vi "Facade - impuls graph.vi"(0 "Data In":T4, 2 "Display State In":T2, 3 "Container State":T3) -> (6 "Data Out":T4, 7 "Display State Out":T2, 8 "Action":T1)   [LabVIEW 2016, in "impuls graph.xctl"]
uses:
  impuls graph.xctl
  Data - impuls graph.ctl
  <vilib>/_xctls/Container State.ctl
  State - impuls graph.ctl
  <vilib>/_xctls/Action.ctl
  <vilib>/_xctls/XControlSupport.lvlib
panel:
  out "Waveform Graph":dbl[][](graph)
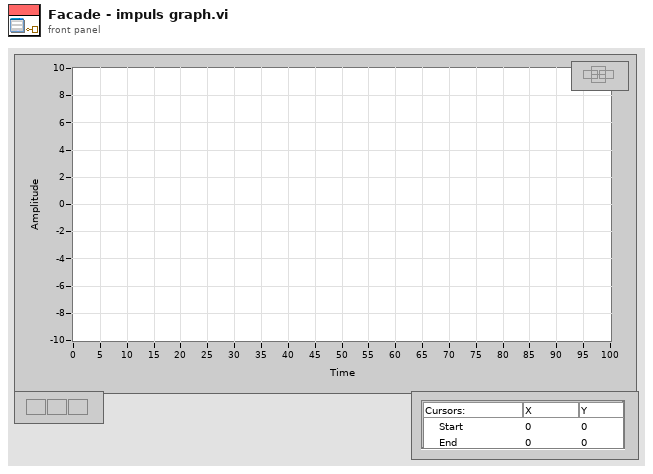
[diagram p1: front panel]
types:
  T1 = typedef "XControlSupport.lvlib/Action.ctl" = cluster{"Data Changed?":bool, "State Changed?":bool, "Action Name":string}
  T2 = typedef "impuls graph.xctl/State - impuls graph.ctl" = cluster{"Waveform Graph":refnum<vi>}
  T3 = typedef "XControlSupport.lvlib/Container State.ctl" = cluster{"Indicator?":bool, "Run Mode?":bool, " Refnum":refnum<vi>}
  T4 = typedef "impuls graph.xctl/Data - impuls graph.ctl" = cluster{"Data":dbl[][], "Colour":u32, "Channel Name":string, "Sample Rate":dbl, "Visible":bool}[]
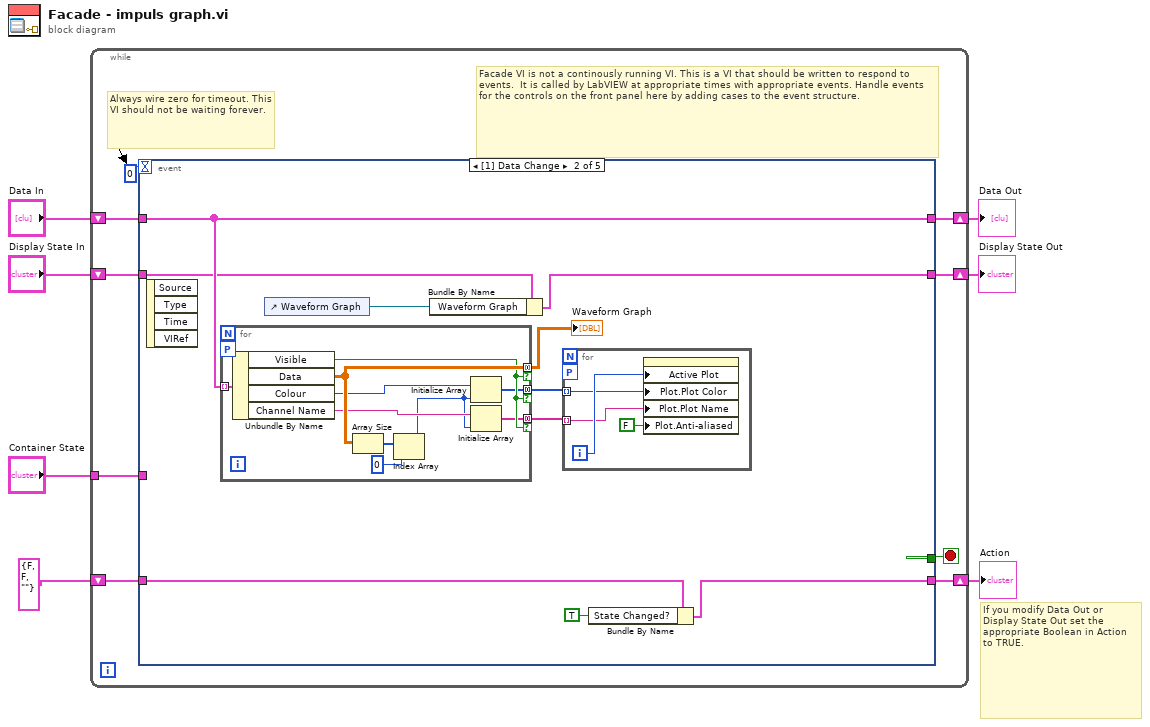
[diagram p0: block diagram]
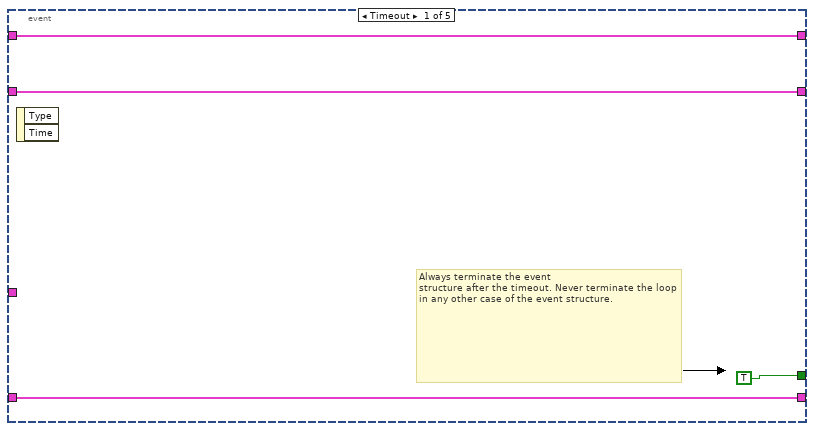
[diagram p2: hidden frame]
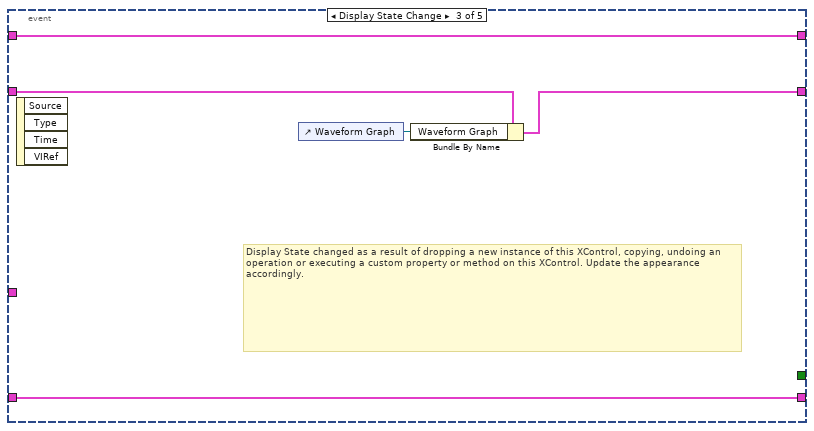
[diagram p3: hidden frame]
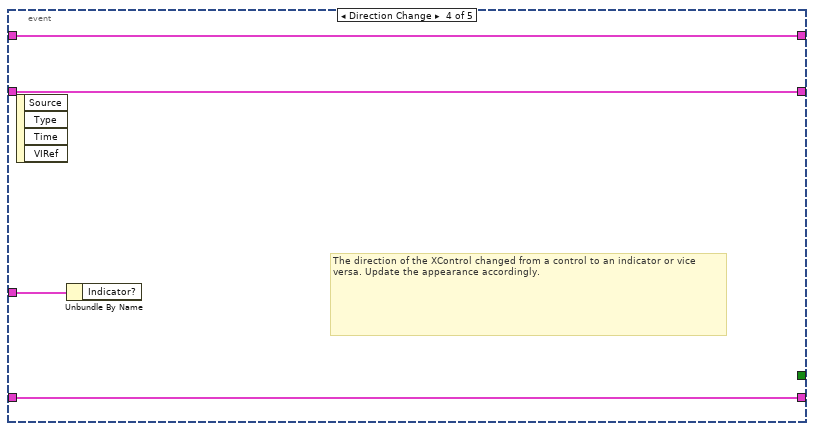
[diagram p4: hidden frame]
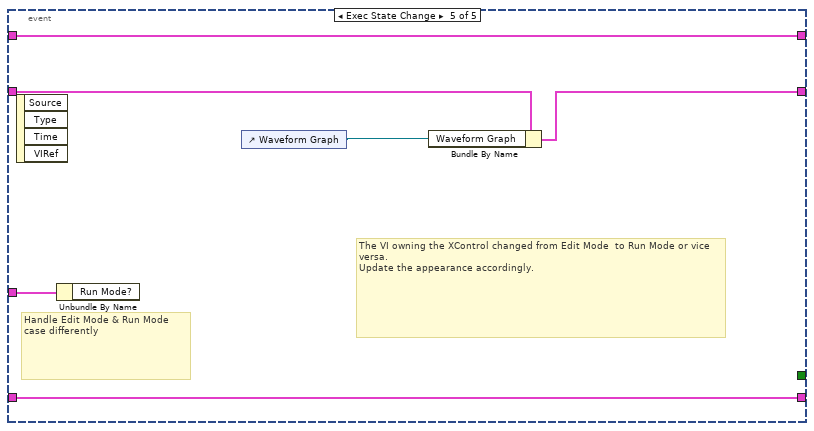
[diagram p5: hidden frame]
diagram:
  # "If you modify Data Out or\nDisplay State Out set the\nappropriate Boolean in Action\nto TRUE."
  n1 = while {
    shift-right: [w15] -> w4
    shift-left: "Display State In" -> [w16]
    tunnel: "Container State" -> [w12]
    shift-right: [w10] -> w7
    shift-left: "Data In" -> [w11]
    shift-right: [w8] -> w2
    shift-left: T1 {"Data Changed?"=FALSE, "State Changed?"=FALSE, "Action Name"=""} ("Action") -> [w9]
    stop <- w14 stop-if-true
    # "Facade VI is not a continously running VI. This is a VI that should be written to respond to events.  It is called by LabVIEW at appropriate times with appropriate events. Handle events for the controls on the front panel here by adding cases to the event structure."
    # "Always wire zero for timeout. This\nVI should not be waiting forever."
    n2 = event shown="[1] Data Change" {
      selector: _ -> [_ _ _ _ _]
      dyn-events: _ -> [_ _ _ _ _]
      timeout: 0 -> [_ _ _ _ _]
      tunnel: w16 -> [w18 w26 w47 w52 w56]
      tunnel: [w18 w25 w46 w52 w55] -> w15
      tunnel: [TRUE _ _ _ _] -> w14
      tunnel: w12 -> [_ _ _ w53 w59]
      tunnel: w11 -> [w17 w30 w49 w51 w58]
      tunnel: [w17 w30 w49 w51 w58] -> w10
      tunnel: [w19 w22 w48 w50 w57] -> w8
      tunnel: w9 -> [w19 w23 w48 w50 w57]
      event Timeout {
        # "Always terminate the event\nstructure after the timeout. Never terminate the loop in any other case of the event structure."
        n3 = event-data() -> ()  [unwired: 1 in, 2 out]
      }
      event Data Change {
        n4 = event-data() -> ()  [unwired: 1 in, 4 out]
        n5 = for {
          tunnel: w30 -> [w44] mode=indexing
          tunnel: [w43] -> w29 mode=concatenating if=w40
          tunnel: [w39] -> w28 mode=concatenating if=w40
          tunnel: [w37] -> w27 mode=concatenating if=w40
          workers-P: _ -> [_]
          n6 = Unbundle By Name(w44) -> ("Visible"=w40:bool, "Data"=w43:dbl[][], "Colour"=w38:u32, "Channel Name"=w36:string)
          n7 = Array Size(array=w43) -> (size(s)=w42:i32[])
          n8 = Index Array(array=w42, index=0) -> (element=w35:i32)
          n9 = Initialize Array(w38, w35) -> (w39:u32[])
          n10 = Initialize Array(w36, w35) -> (w37:string[])
        }
        "Waveform Graph" <- w29
        n11 = control-ref of="Waveform Graph"() -> (w24:refnum<vi>)
        n12 = Bundle By Name(cluster=w26, "Waveform Graph"=w24) -> (w25:T2)
        n13 = for {
          tunnel: w28 -> [w33] mode=indexing
          tunnel: w27 -> [w32] mode=indexing
          workers-P: _ -> [_]
          i -> [w34]
          n14 = property on="Waveform Graph" class="WFGraph (strict)"("Active Plot"=w34, "Plot.Plot Color"=w33, "Plot.Plot Name"=w32, "Plot.Anti-aliased"=FALSE) -> ()  [unwired: 2 in, 2 out]
        }
        n15 = Bundle By Name(cluster=w23, "State Changed?"=TRUE) -> (w22:T1)
      }
      event Display State Change {
        # "Display State changed as a result of dropping a new instance of this XControl, copying, undoing an operation or executing a custom property or method on this XControl. Update the appearance accordingly."
        n16 = event-data() -> ()  [unwired: 1 in, 4 out]
        n17 = control-ref of="Waveform Graph"() -> (w45:refnum<vi>)
        n18 = Bundle By Name(cluster=w47, "Waveform Graph"=w45) -> (w46:T2)
      }
      event Direction Change {
        # "The direction of the XControl changed from a control to an indicator or vice versa. Update the appearance accordingly."
        n19 = event-data() -> ()  [unwired: 1 in, 4 out]
        n20 = Unbundle By Name(w53) -> ()  [unwired: 1 out]
      }
      event Exec State Change {
        # "The VI owning the XControl changed from Edit Mode  to Run Mode or vice versa.\nUpdate the appearance accordingly."
        # "Handle Edit Mode & Run Mode\ncase differently"
        n21 = event-data() -> ()  [unwired: 1 in, 4 out]
        n22 = Unbundle By Name(w59) -> ()  [unwired: 1 out]
        n23 = control-ref of="Waveform Graph"() -> (w54:refnum<vi>)
        n24 = Bundle By Name(cluster=w56, "Waveform Graph"=w54) -> (w55:T2)
      }
    }
  }
  "Display State Out" <- w4
  "Data Out" <- w7
  "Action" <- w2
